vi "UI Main.vi"() -> ()   [LabVIEW 2020]
uses:
  controls/Control Configuration.ctl
  controls/UI Data.ctl
  controls/All Control Configuration Values.ctl
  controls/Control State.ctl
  controls/Raw Values.ctl
  Globals/Global - All UI Loop Stop.vi
  Globals/Global - UI Stream and Variable Connections.vi
  Globals/Global - Configuration Options.vi
  support/User Event - Stop/User Event - Stop.lvlib
  support/Message Queue/Message Queue.lvlib
panel:
  in  "Switch to Safe State":bool
  in  "Exit":bool
  out "System Status":string
  out "Current Control Mode":u16(ring) items=["Safe State", "Manual", "Control (PID)"]
  in  "Settings Tab":T1(tab)
  in  "Channel 3 Setpoint":dbl
  in  "Channel 2 Setpoint":dbl
  in  "Channel 1 Setpoint":dbl
  in  "Channel 0 Setpoint":dbl
  in  "Update Control Configuration":bool
  in  "Control Configurations":T2[](array[typedef])
  in  "Run Control":bool
  in  "Stop Control":bool
  in  "Channel 3 Manual Value":dbl
  in  "Channel 2 Manual Value":dbl
  in  "Channel 1 Manual Value":dbl
  in  "Channel 0 Manual Value":dbl
  in  "Run Manual":bool
  in  "Stop Manual":bool
  out "Control Input Values":T3(graph)
  out "Control Output Values":T3(graph)
  out "Control Loop Period (ms)":u32
  out "Largest Contiguous Memory (bytes)":dbl(graph)
  out "CPU Usage (%)":dbl(graph)
  out "Connected?":bool
  in  "Connect to Controller":bool
  in  "Controller Address":string
  # "LabVIEW Real-Time Control (NI-DAQmx)"
  # "Connection Settings"
  # "Element 0 - Chan 0\nElement 1 - Chan 1\nElement 2 - Chan 2\nElement 3 - Chan 3"
  # "Setpoint changes are sent to the target automatically."
  # "Control Configuration changes are sent to the target when you click \"Update Control Configurations\"."
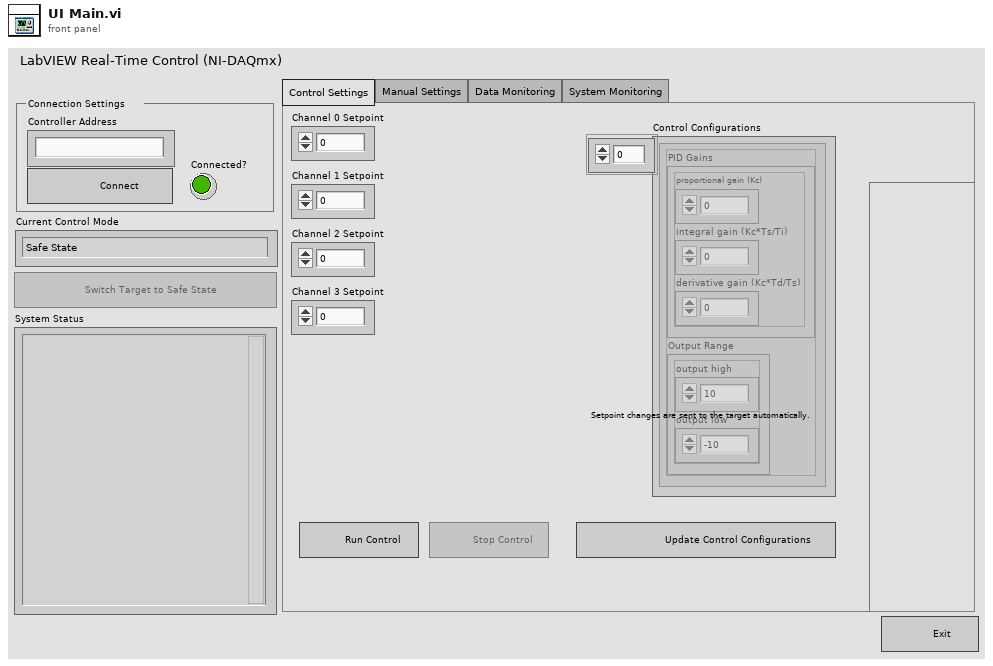
[diagram p1: front panel]
types:
  T1 = enum32{"Control Settings", "Manual Settings", "Data Monitoring", "System Monitoring"}
  T2 = typedef "Control Configuration.ctl" = cluster{"PID Gains":cluster{"proportional gain (Kc)":dbl, "integral gain (Kc*Ts/Ti)":dbl, "derivative gain (Kc*Td/Ts)":dbl}, "Output Range":cluster{"output high":dbl, "output low":dbl}}
  T3 = cluster{"Array of Double[0]":dbl, "Array of Double[1]":dbl, "Array of Double[2]":dbl, "Array of Double[3]":dbl}
  T4 = typedef "UI Data.ctl" = cluster{"Switch to Safe State Ref":refnum<vi>, "Run Manual Ref":refnum<vi>, "Stop Manual Ref":refnum<vi>, "Run Control Ref":refnum<vi>, "Stop Control Ref":refnum<vi>, "Update Control Configurations Ref":refnum<vi>, "Ch 0 Setpoint Ref":refnum<vi>, "Ch 1 Setpoint Ref":refnum<vi>, "Ch 2 Setpoint Ref":refnum<vi>, "Ch 3 Setpoint Ref":refnum<vi>, "Ch 0 Manual Ref":refnum<vi>, "Ch 1 Manual Ref":refnum<vi>, "Ch 2 Manual Ref":refnum<vi>, "Ch 3 Manual Ref":refnum<vi>, "Control Configurations Ref":refnum<vi>}
  T5 = typedef "Message Queue.lvlib/All Message Queues.ctl" = cluster{"UI":refnum<queue>}
  T6 = typedef "Variable References.ctl" = cluster{"CPU Usage":refnum<k21>, "Contiguous Memory":refnum<k21>, "Control Mode":refnum<k21>, "Control Loop Period":refnum<k21>, "Input Values":refnum<k21>, "Output Values":refnum<k21>}
  T7 = typedef "Control State.ctl" = enum16{"Safe State", "Manual", "Control (PID)"}
  T8 = cluster{"Channel 0 Setpoint":dbl, "Channel 1 Setpoint":dbl, "Channel 2 Setpoint":dbl, "Channel 3 Setpoint":dbl}
  T9 = cluster{"Channel 0 Manual Value":dbl, "Channel 1 Manual Value":dbl, "Channel 2 Manual Value":dbl, "Channel 3 Manual Value":dbl}
  T10 = cluster{"Message":string, "Message Data":variant}
  T11 = typedef "All Control Configuration Values.ctl" = cluster{"Control State":T7, "Setpoints":T12, "Manual Values":T12, "Control Configurations":T2[]}
  T12 = typedef "Raw Values.ctl" = cluster{"Channel 0":dbl, "Channel 1":dbl, "Channel 2":dbl, "Channel 3":dbl}
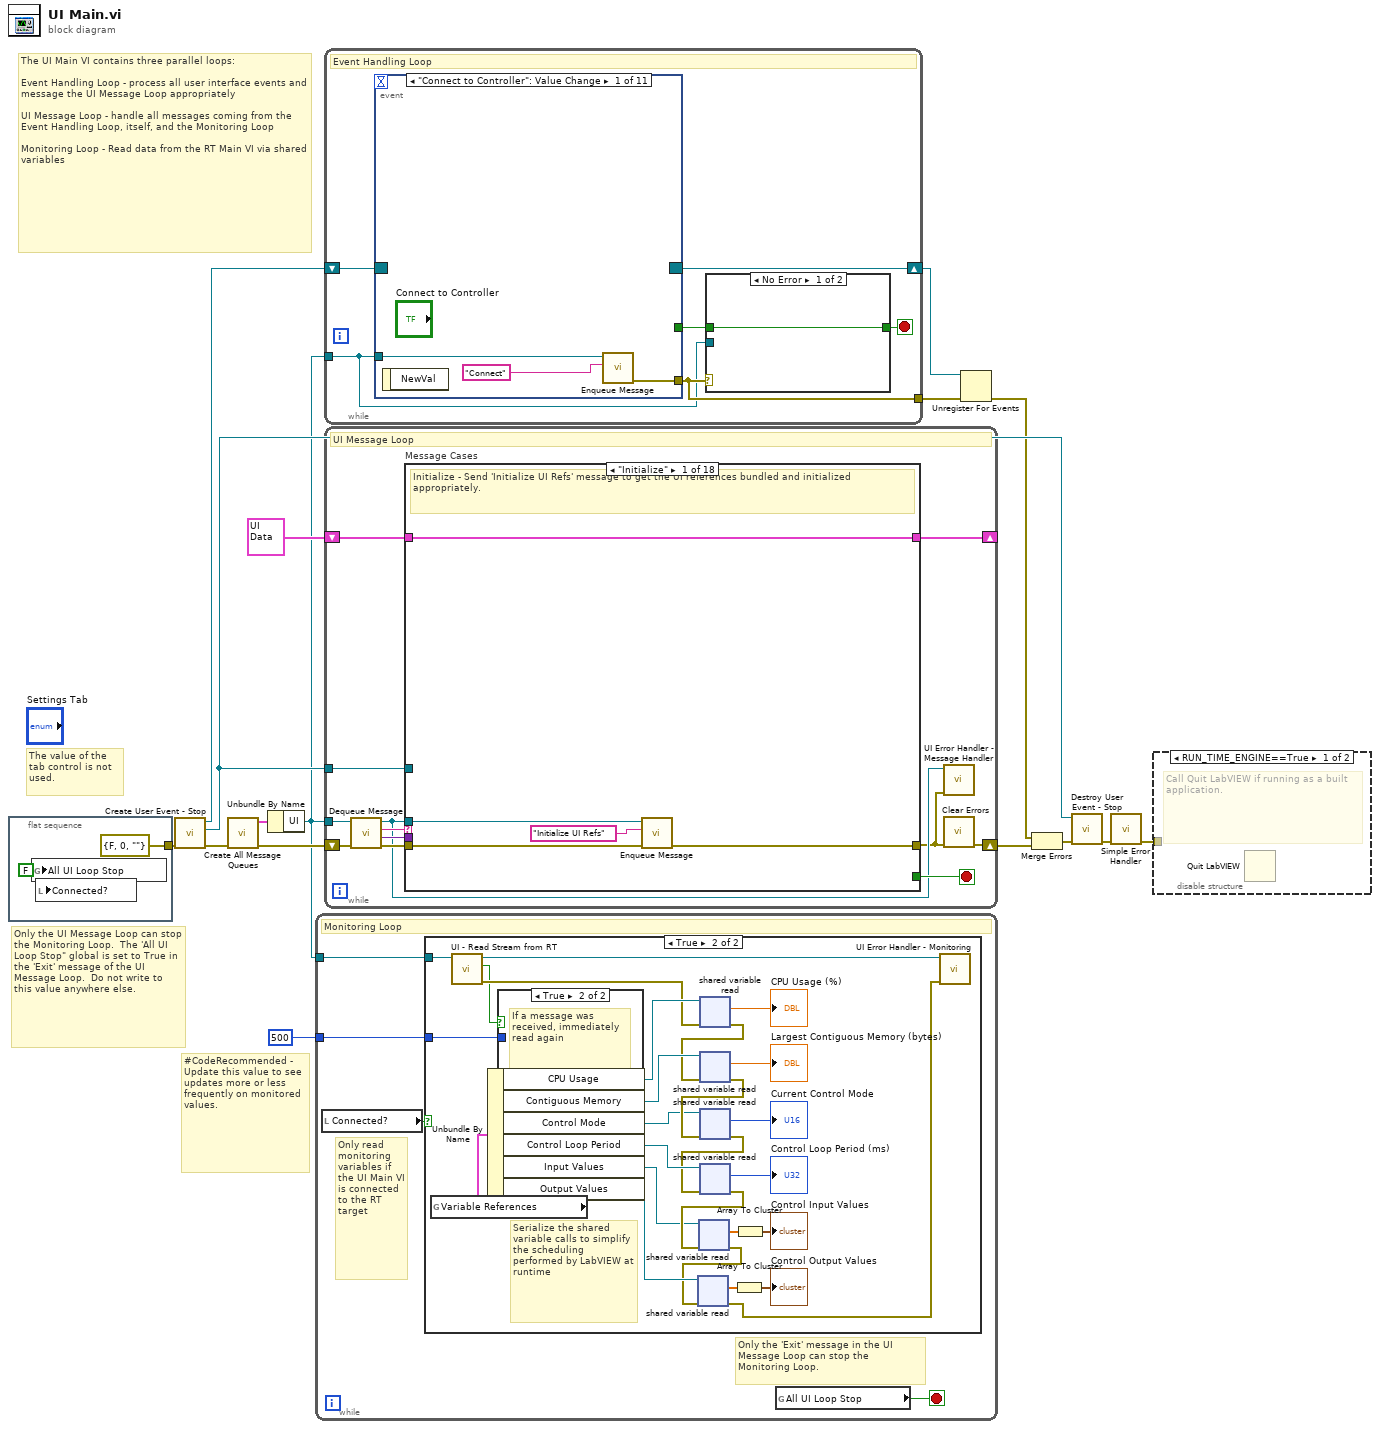
[diagram p0: block diagram]
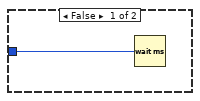
[diagram p3: hidden frame]
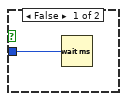
[diagram p4: hidden frame]
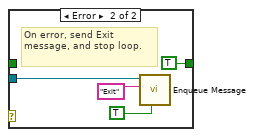
[diagram p5: hidden frame]
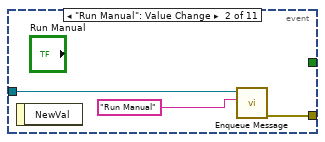
[diagram p6: hidden frame]
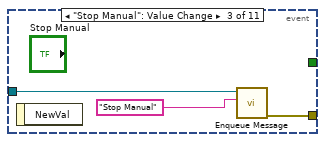
[diagram p7: hidden frame]
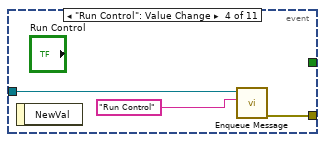
[diagram p8: hidden frame]
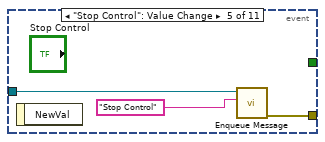
[diagram p9: hidden frame]
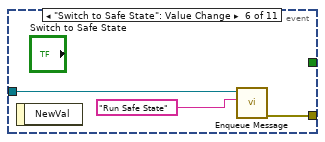
[diagram p10: hidden frame]
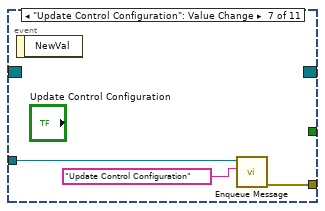
[diagram p11: hidden frame]
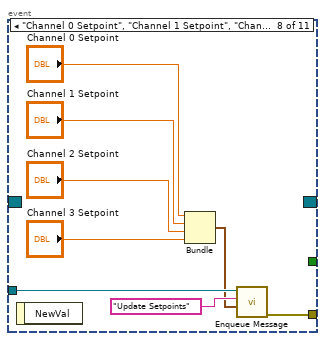
[diagram p12: hidden frame]
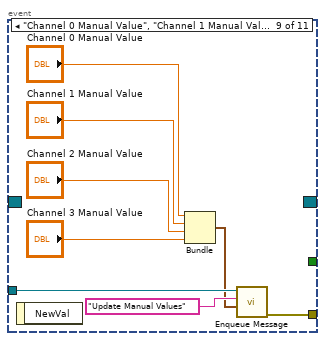
[diagram p13: hidden frame]
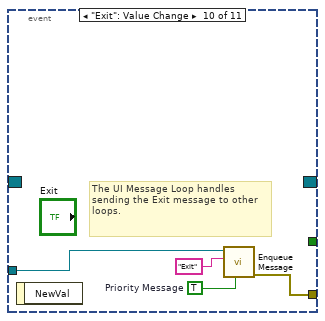
[diagram p14: hidden frame]
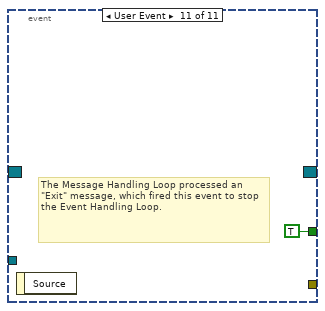
[diagram p15: hidden frame]
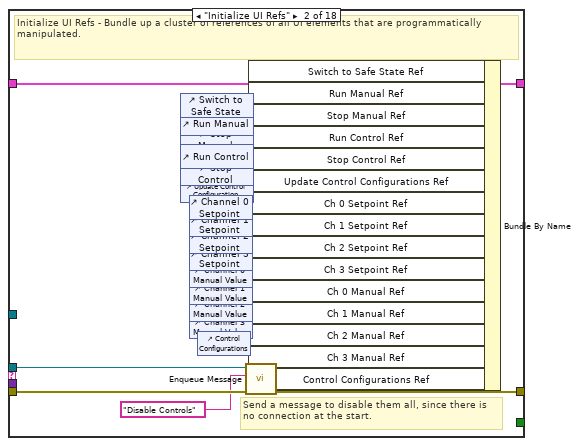
[diagram p16: hidden frame]
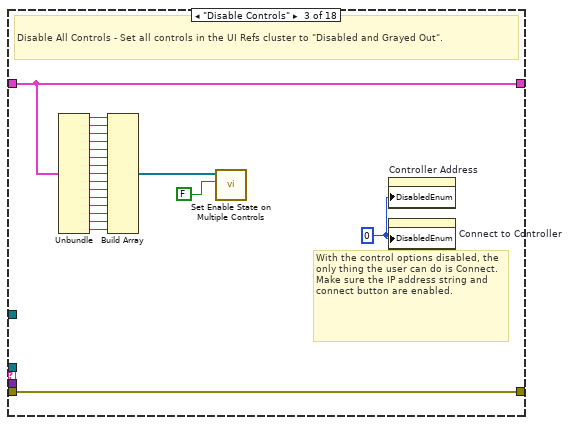
[diagram p17: hidden frame]
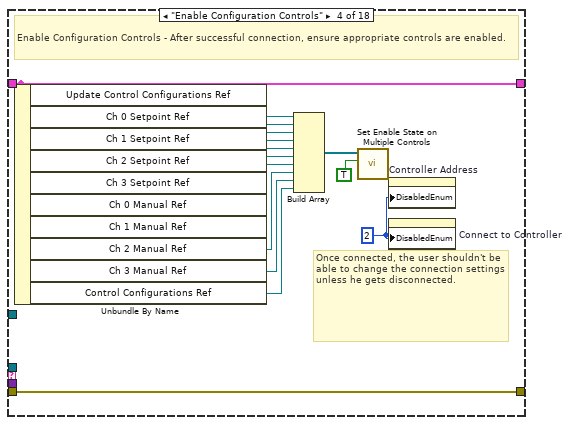
[diagram p18: hidden frame]
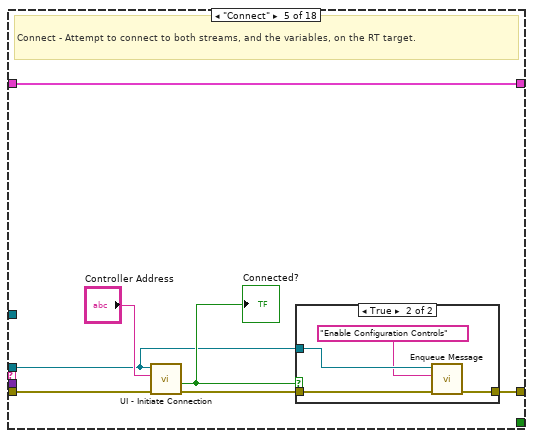
[diagram p19: hidden frame]
diagram:
  # "#CodeRecommended - Update this value to see updates more or less frequently on monitored values."
  # "The UI Main VI contains three parallel loops:\n\nEvent Handling Loop - process all user interface events and message the UI Message Loop appropriately\n\nUI Message Loop - handle all messages coming from the Event Handling Loop, itself, and the Monitoring Loop\n\nMonitoring Loop - Read data from the RT Main VI via shared variables"
  # "The value of the tab control is not used."
  # "Only the UI Message Loop can stop the Monitoring Loop.  The 'All UI Loop Stop\" global is set to True in the 'Exit' message of the UI Message Loop.  Do not write to this value anywhere else."
  n1 = flat-sequence {
    tunnel: [errorcluster {"status"=FALSE, "code"=0, "source"=""} ("error in (no error)")] -> w3
    frame #0 {
      w17 = FALSE
      n2 = global write "Global - All UI Loop Stop.vi" "All UI Loop Stop"(w17) -> ()
      n3 = local write "Connected?"(w17) -> ()
    }
  }
  n4 = call "Create User Event - Stop.vi"("error in (no error)"=w3) -> ("error out"=w11:errorcluster, "User Event - Stop"=w12:refnum<user-event>, "Stop Event Registration Refnum"=w13:refnum<event-registration>)  [unwired: 8 in]
  n5 = call "Create All Message Queues.vi"("error in (no error)"=w11) -> ("error out"=w9:errorcluster, "Message Queues out"=w10:T5)  [unwired: 9 in]
  n6 = Unbundle By Name(w10) -> ("UI"=w4:refnum<queue>)
  n7 = while {
    tunnel: w4 -> [w21]
    tunnel: u32 500 ("milliseconds to wait") -> [w19]
    stop <- w22 stop-if-true
    # "Only read monitoring variables if the UI Main VI is connected to the RT target"
    # "Only the 'Exit' message in the UI Message Loop can stop the Monitoring Loop."
    # "Monitoring Loop"
    n8 = local read "Connected?"() -> (w20:bool)
    n9 = case shown="True" w20 {
      tunnel: w21 -> [_ w40]
      tunnel: w19 -> [w23 w35]
      frame False {
        n10 = Wait (ms)(milliseconds to wait=w23) -> ()  [unwired: 1 out]
      }
      frame True {
        # "Serialize the shared variable calls to simplify the scheduling performed by LabVIEW at runtime"
        n11 = global read "Global - UI Stream and Variable Connections.vi" "Variable References"() -> (w38:T6)
        n12 = call "UI - Read Stream from RT.vi"("Message Queue"=w40) -> ("error out"=w43:errorcluster, "Message Received?"=w36:bool, "dup Message Queue"=w39:refnum<queue>)  [unwired: 8 in]
        n13 = Unbundle By Name(w38) -> ("CPU Usage"=w46:refnum<k21>, "Contiguous Memory"=w45:refnum<k21>, "Control Mode"=w33:refnum<k21>, "Control Loop Period"=w44:refnum<k21>, "Input Values"=w31:refnum<k21>, "Output Values"=w29:refnum<k21>)
        n14 = case shown="True" w36 {
          tunnel: w35 -> [w50 _]
          frame False {
            n15 = Wait (ms)(milliseconds to wait=w50) -> ()  [unwired: 1 out]
          }
          frame True {
            # "If a message was received, immediately read again"
          }
        }
        n16 = shared-variable-read(w46, w43) -> (w42:errorcluster, →"CPU Usage (%)":dbl)  [unwired: 2 out]
        n17 = shared-variable-read(w45, w42) -> (w34:errorcluster, →"Largest Contiguous Memory (bytes)":dbl)  [unwired: 2 out]
        n18 = shared-variable-read(w33, w34) -> (w41:errorcluster, →"Current Control Mode":T7)  [unwired: 2 out]
        n19 = shared-variable-read(w44, w41) -> (w32:errorcluster, →"Control Loop Period (ms)":u32)  [unwired: 2 out]
        n20 = shared-variable-read(w31, w32) -> (w28:errorcluster, w30:dbl[])  [unwired: 2 out]
        n21 = shared-variable-read(w29, w28) -> (w26:errorcluster, w27:dbl[])  [unwired: 2 out]
        n22 = Array To Cluster(array=w27) -> (cluster=→"Control Output Values":T3)
        n23 = Array To Cluster(array=w30) -> (cluster=→"Control Input Values":T3)
        n24 = call "UI Error Handler - Monitoring.vi"("error in (no error)"=w26, "Message Queue"=w39) -> ()  [unwired: 9 in, 1 out]
      }
    }
    n25 = global read "Global - All UI Loop Stop.vi" "All UI Loop Stop"() -> (w22:bool)
  }
  n26 = while {
    tunnel: w4 -> [w52]
    tunnel: [w54] -> w15
    shift-right: [w51] -> w7
    shift-left: w13 -> [w53]
    stop <- w55 stop-if-true
    # "Event Handling Loop"
    n27 = event shown="[0] \"Connect to Controller\": Value Change" {
      selector: w53 -> [_ _ _ _ _ _ _ _ _ _ _]
      dyn-events: [_ _ _ _ _ _ _ _ _ _ _] -> w51
      timeout: _ -> [_ _ _ _ _ _ _ _ _ _ _]
      tunnel: [_ _ _ _ _ _ _ _ _ _ TRUE ("Discard?")] -> w56
      tunnel: w52 -> [w62 w65 w68 w71 w74 w77 w82 w85 w97 w99 _]
      tunnel: [w64 w67 w70 w73 w76 w79 w81 w84 w96 w102 _] -> w54
      event "Connect to Controller": Value Change {
        n28 = event-data() -> ()  [unwired: 1 in, 1 out]
        n29 = call "Enqueue Message.vi"("Message"="Connect", "Message Queue"=w62) -> ("error out"=w64:errorcluster)  [unwired: 8 in, 1 out]
      }
      event "Run Manual": Value Change {
        n30 = event-data() -> ()  [unwired: 1 in, 1 out]
        n31 = call "Enqueue Message.vi"("Message"="Run Manual", "Message Queue"=w65) -> ("error out"=w67:errorcluster)  [unwired: 8 in, 1 out]
      }
      event "Stop Manual": Value Change {
        n32 = event-data() -> ()  [unwired: 1 in, 1 out]
        n33 = call "Enqueue Message.vi"("Message"="Stop Manual", "Message Queue"=w68) -> ("error out"=w70:errorcluster)  [unwired: 8 in, 1 out]
      }
      event "Run Control": Value Change {
        n34 = event-data() -> ()  [unwired: 1 in, 1 out]
        n35 = call "Enqueue Message.vi"("Message"="Run Control", "Message Queue"=w71) -> ("error out"=w73:errorcluster)  [unwired: 8 in, 1 out]
      }
      event "Stop Control": Value Change {
        n36 = event-data() -> ()  [unwired: 1 in, 1 out]
        n37 = call "Enqueue Message.vi"("Message"="Stop Control", "Message Queue"=w74) -> ("error out"=w76:errorcluster)  [unwired: 8 in, 1 out]
      }
      event "Switch to Safe State": Value Change {
        n38 = event-data() -> ()  [unwired: 1 in, 1 out]
        n39 = call "Enqueue Message.vi"("Message"="Run Safe State", "Message Queue"=w77) -> ("error out"=w79:errorcluster)  [unwired: 8 in, 1 out]
      }
      event "Update Control Configuration": Value Change {
        n40 = event-data() -> ()  [unwired: 1 in, 1 out]
        n41 = call "Enqueue Message.vi"("Message"="Update Control Configuration", "Message Queue"=w82) -> ("error out"=w81:errorcluster)  [unwired: 8 in, 1 out]
      }
      event "Channel 0 Setpoint", "Channel 1 Setpoint", "Channel 2 Setpoint", "Channel 3 Setpoint": Value Change {
        n42 = event-data() -> ()  [unwired: 1 in, 1 out]
        n43 = Bundle("Channel 0 Setpoint"="Channel 0 Setpoint", "Channel 1 Setpoint"="Channel 1 Setpoint", "Channel 2 Setpoint"="Channel 2 Setpoint", "Channel 3 Setpoint"="Channel 3 Setpoint") -> (w83:T8)  [unwired: 1 in]
        n44 = call "Enqueue Message.vi"("Message Data"=w83, "Message"="Update Setpoints", "Message Queue"=w85) -> ("error out"=w84:errorcluster)  [unwired: 7 in, 1 out]
      }
      event "Channel 0 Manual Value", "Channel 1 Manual Value", "Channel 2 Manual Value", "Channel 3 Manual Value": Value Change {
        n45 = event-data() -> ()  [unwired: 1 in, 1 out]
        n46 = Bundle("Channel 0 Manual Value"="Channel 0 Manual Value", "Channel 1 Manual Value"="Channel 1 Manual Value", "Channel 2 Manual Value"="Channel 2 Manual Value", "Channel 3 Manual Value"="Channel 3 Manual Value") -> (w95:T9)  [unwired: 1 in]
        n47 = call "Enqueue Message.vi"("Message Data"=w95, "Message"="Update Manual Values", "Message Queue"=w97) -> ("error out"=w96:errorcluster)  [unwired: 7 in, 1 out]
      }
      event "Exit": Value Change {
        w100 = TRUE  # Priority Message
        # "The UI Message Loop handles sending the Exit message to other loops."
        n48 = event-data() -> ()  [unwired: 1 in, 1 out]
        n49 = call "Enqueue Message.vi"("Priority Message? (F)"=w100, "Message"="Exit", "Message Queue"=w99) -> ("error out"=w102:errorcluster)  [unwired: 7 in, 1 out]
      }
      event User Event {
        # "The Message Handling Loop processed an \"Exit\" message, which fired this event to stop the Event Handling Loop."
        n50 = event-data() -> ()  [unwired: 1 in, 1 out]
      }
    }
    n51 = case shown="No Error" w54 {
      tunnel: [w57 TRUE ("Discard?")] -> w55
      tunnel: w56 -> [w57 _]
      tunnel: w52 -> [_ w58]
      frame No Error {
      }
      frame Error {
        # "On error, send Exit message, and stop loop."
        n52 = call "Enqueue Message.vi"("Priority Message? (F)"=TRUE ("Discard?"), "Message"="Exit", "Message Queue"=w58) -> ()  [unwired: 7 in, 2 out]
      }
    }
  }
  n53 = while {
    tunnel: w4 -> [w109]
    tunnel: w12 -> [w114]
    shift-right: [w104] -> w16
    shift-left: w9 -> [w113]
    shift-right: [w107] -> _
    shift-left: T4 {"Switch to Safe State Ref"=refnum, "Run Manual Ref"=refnum, "Stop Manual Ref"=refnum, "Run Control Ref"=refnum, "Stop Control Ref"=refnum, "Update Control Configurations Ref"=refnum, "Ch 0 Setpoint Ref"=refnum, "Ch 1 Setpoint Ref"=refnum, "Ch 2 Setpoint Ref"=refnum, "Ch 3 Setpoint Ref"=refnum, "Ch 0 Manual Ref"=refnum, "Ch 1 Manual Ref"=refnum, "Ch 2 Manual Ref"=refnum, "Ch 3 Manual Ref"=refnum, "Control Configurations Ref"=refnum} ("Measurement UI Controls") -> [w108]
    stop <- w115 stop-if-true
    # "UI Message Loop"
    n54 = call "Dequeue Message.vi"("error in (no error)"=w113, "Message Queue"=w109) -> ("error out"=w112:errorcluster, "Message Data"=w110:variant, "Message"=w111:string, "dup Message Queue"=w106:refnum<queue>)  [unwired: 6 in]
    n55 = case "Message Cases" shown="\"Initialize\"" w111 {
      selector: w111 -> [_ _ _ _ _ _ _ _ _ w238 _ w270 _ w320 _ _ _ w382]
      tunnel: w106 -> [w117 w129 _ _ w178 _ w196 _ w220 w239 _ _ _ w324 _ w367 _ _]
      tunnel: w112 -> [w119 w141 w161 w167 w183 w194 w198 w203 w234 w241 w259 w271 w284 w334 w355 w372 w377 _]
      tunnel: [w118 w130 w161 w167 w177 w194 w197 w202 w222 w240 w258 w272 w282 w335 w353 w373 w376 w380] -> w105
      tunnel: [_ _ _ _ _ _ _ _ _ _ _ _ _ _ _ TRUE _ _] -> w115
      tunnel: w110 -> [_ _ _ _ _ _ _ _ w232 _ _ w269 w283 w332 w352 _ _ _]
      tunnel: w114 -> [_ _ _ _ _ _ _ _ _ _ _ _ _ _ _ w371 _ _]
      tunnel: w108 -> [w120 w140 w160 w173 w182 w193 w200 w204 w229 w242 w260 w273 w281 w336 w354 w369 w375 w378]
      tunnel: [w120 w139 w160 w173 w182 w193 w200 w204 w229 w242 w260 w273 w281 w336 w354 w369 w375 w378] -> w107
      frame "Initialize" {
        # "Initialize - Send 'Initialize UI Refs' message to get the UI references bundled and initialized appropriately."
        n56 = call "Enqueue Message.vi"("error in (no error)"=w119, "Message"="Initialize UI Refs", "Message Queue"=w117) -> ("error out"=w118:errorcluster)  [unwired: 7 in, 1 out]
      }
      frame "Initialize UI Refs" {
        # "Send a message to disable them all, since there is no connection at the start."
        # "Initialize UI Refs - Bundle up a cluster of references of all UI elements that are programmatically manipulated."
        n57 = control-ref of="Switch to Safe State"() -> (w138:refnum<vi>)
        n58 = control-ref of="Run Manual"() -> (w122:refnum<vi>)
        n59 = control-ref of="Stop Manual"() -> (w121:refnum<vi>)
        n60 = control-ref of="Run Control"() -> (w137:refnum<vi>)
        n61 = control-ref of="Stop Control"() -> (w136:refnum<vi>)
        n62 = control-ref of="Update Control Configuration"() -> (w135:refnum<vi>)
        n63 = control-ref of="Channel 0 Setpoint"() -> (w134:refnum<vi>)
        n64 = control-ref of="Channel 1 Setpoint"() -> (w133:refnum<vi>)
        n65 = control-ref of="Channel 2 Setpoint"() -> (w132:refnum<vi>)
        n66 = control-ref of="Channel 3 Setpoint"() -> (w131:refnum<vi>)
        n67 = control-ref of="Channel 0 Manual Value"() -> (w126:refnum<vi>)
        n68 = control-ref of="Channel 1 Manual Value"() -> (w125:refnum<vi>)
        n69 = control-ref of="Channel 2 Manual Value"() -> (w124:refnum<vi>)
        n70 = control-ref of="Channel 3 Manual Value"() -> (w123:refnum<vi>)
        n71 = control-ref of="Control Configurations"() -> (w127:refnum<vi>)
        n72 = call "Enqueue Message.vi"("error in (no error)"=w141, "Message"="Disable Controls", "Message Queue"=w129) -> ("error out"=w130:errorcluster)  [unwired: 7 in, 1 out]
        n73 = Bundle By Name(cluster=w140, "Switch to Safe State Ref"=w138, "Run Manual Ref"=w122, "Stop Manual Ref"=w121, "Run Control Ref"=w137, "Stop Control Ref"=w136, "Update Control Configurations Ref"=w135, "Ch 0 Setpoint Ref"=w134, "Ch 1 Setpoint Ref"=w133, "Ch 2 Setpoint Ref"=w132, "Ch 3 Setpoint Ref"=w131, "Ch 0 Manual Ref"=w126, "Ch 1 Manual Ref"=w125, "Ch 2 Manual Ref"=w124, "Ch 3 Manual Ref"=w123, "Control Configurations Ref"=w127) -> (w139:T4)
      }
      frame "Disable Controls" {
        w148 = 0
        # "With the control options disabled, the only thing the user can do is Connect. Make sure the IP address string and connect button are enabled."
        # "Disable All Controls - Set all controls in the UI Refs cluster to \"Disabled and Grayed Out\"."
        n74 = Unbundle(w160) -> ("Switch to Safe State Ref"=w159:refnum<vi>, "Run Manual Ref"=w158:refnum<vi>, "Stop Manual Ref"=w157:refnum<vi>, "Run Control Ref"=w156:refnum<vi>, "Stop Control Ref"=w155:refnum<vi>, "Update Control Configurations Ref"=w154:refnum<vi>, "Ch 0 Setpoint Ref"=w153:refnum<vi>, "Ch 1 Setpoint Ref"=w152:refnum<vi>, "Ch 2 Setpoint Ref"=w151:refnum<vi>, "Ch 3 Setpoint Ref"=w147:refnum<vi>, "Ch 0 Manual Ref"=w146:refnum<vi>, "Ch 1 Manual Ref"=w145:refnum<vi>, "Ch 2 Manual Ref"=w144:refnum<vi>, "Ch 3 Manual Ref"=w143:refnum<vi>, "Control Configurations Ref"=w142:refnum<vi>)
        n75 = Build Array(w159, w158, w157, w156, w155, w154, w153, w152, w151, w147, w146, w145, w144, w143, w142) -> (w150:refnum<vi>[])
        n76 = call "Set Enable State on Multiple Controls.vi"("Enable?"=FALSE, "Controls"=w150) -> ()  [unwired: 10 in]
        n77 = property on="Controller Address" class="Str"("DisabledEnum"=w148) -> ()  [unwired: 2 in, 2 out]
        n78 = property on="Connect to Controller" class="Bool"("DisabledEnum"=w148) -> ()  [unwired: 2 in, 2 out]
      }
      frame "Enable Configuration Controls" {
        w174 = 2
        # "Once connected, the user shouldn't be able to change the connection settings unless he gets disconnected."
        # "Enable Configuration Controls - After successful connection, ensure appropriate controls are enabled."
        n79 = Unbundle By Name(w173) -> ("Update Control Configurations Ref"=w172:refnum<vi>, "Ch 0 Setpoint Ref"=w171:refnum<vi>, "Ch 1 Setpoint Ref"=w170:refnum<vi>, "Ch 2 Setpoint Ref"=w169:refnum<vi>, "Ch 3 Setpoint Ref"=w168:refnum<vi>, "Ch 0 Manual Ref"=w166:refnum<vi>, "Ch 1 Manual Ref"=w165:refnum<vi>, "Ch 2 Manual Ref"=w164:refnum<vi>, "Ch 3 Manual Ref"=w163:refnum<vi>, "Control Configurations Ref"=w162:refnum<vi>)
        n80 = Build Array(w172, w171, w170, w169, w168, w166, w165, w164, w163, w162) -> (w176:refnum<vi>[])
        n81 = call "Set Enable State on Multiple Controls.vi"("Enable?"=TRUE, "Controls"=w176) -> ()  [unwired: 10 in]
        n82 = property on="Controller Address" class="Str"("DisabledEnum"=w174) -> ()  [unwired: 2 in, 2 out]
        n83 = property on="Connect to Controller" class="Bool"("DisabledEnum"=w174) -> ()  [unwired: 2 in, 2 out]
      }
      frame "Connect" {
        # "Connect - Attempt to connect to both streams, and the variables, on the RT target."
        n84 = call "UI - Initiate Connection.vi"("error in (no error)"=w183, "Controller Address"="Controller Address", "Message Queue"=w178) -> ("error out"=w180:errorcluster, "Connected?"=w179:bool)  [unwired: 7 in]
        "Connected?" <- w179
        n85 = case shown="True" w179 {
          tunnel: w180 -> [w184 w188]
          tunnel: w178 -> [_ w187]
          tunnel: [w184 w186] -> w177
          frame False {
          }
          frame True {
            n86 = call "Enqueue Message.vi"("error in (no error)"=w188, "Message"="Enable Configuration Controls", "Message Queue"=w187) -> ("error out"=w186:errorcluster)  [unwired: 7 in, 1 out]
          }
        }
      }
      frame "Close Connections" {
        # "Close Connections - Close the connections shared with the Monitoring Loop."
        n87 = global read "Global - UI Stream and Variable Connections.vi" "UI Command Stream"() -> (w192:refnum<k21>)
        n88 = global read "Global - UI Stream and Variable Connections.vi" "Variable References"() -> (w190:T6)
        n89 = global read "Global - UI Stream and Variable Connections.vi" "RT Message Stream"() -> (w191:refnum<k21>)
        n90 = local write "Connected?"(FALSE ("Connected?")) -> ()
        n91 = Destroy Stream Endpoint(11:w192) -> ()  [unwired: 1 in, 1 out]
        n92 = Destroy Stream Endpoint(11:w191) -> ()  [unwired: 1 in, 1 out]
        n93 = call "Close Variable Connections.vi"("Variable References"=w190) -> ()  [unwired: 11 in]
      }
      frame "Disconnect UI" {
        # "Disconnect UI - Something has gone wrong with the connection. Reinitialize the UI to its disconnected state."
        n94 = local write "Connected?"(FALSE ("Connected?")) -> ()
        n95 = call "Enqueue Message.vi"("error in (no error)"=w198, "Message"="Disable Controls", "Message Queue"=w196) -> ("error out"=w197:errorcluster)  [unwired: 7 in, 1 out]
      }
      frame "Get Control Settings from RT" {
        # "Get Control Settings from RT - Send a command to the RT to retrieve all current control parameter values and send them back to the UI."
        n96 = local read "Connected?"() -> (w201:bool)
        n97 = case shown="True" w201 {
          tunnel: w203 -> [w205 w209]
          tunnel: [w205 w208] -> w202
          frame False {
            # "Don't bother trying to send a message to the RT system if UI Main VI isn't even connected"
          }
          frame True {
            n98 = global read "Global - UI Stream and Variable Connections.vi" "UI Command Stream"() -> (w206:refnum<k21>)
            n99 = shared-variable-write(w206, w209, T10 {"Message"="Send Control Configuration to UI", "Message Data"=variant} ("data in")) -> (w208:errorcluster)  [unwired: 1 in, 2 out]
          }
        }
      }
      frame "Initial UI Values" {
        # "Set values of all setpoint and manual controls via reference."
        # "Initial UI Values - These are the current control values from the RT Control Loop. They are used to initialize the panel of UI Main VI upon successful connection to the RT target."
        n100 = Unbundle By Name(w229) -> ("Ch 0 Setpoint Ref"=w228:refnum<vi>, "Ch 1 Setpoint Ref"=w227:refnum<vi>, "Ch 2 Setpoint Ref"=w226:refnum<vi>, "Ch 3 Setpoint Ref"=w225:refnum<vi>, "Ch 0 Manual Ref"=w218:refnum<vi>, "Ch 1 Manual Ref"=w217:refnum<vi>, "Ch 2 Manual Ref"=w216:refnum<vi>, "Ch 3 Manual Ref"=w215:refnum<vi>)
        n101 = Variant To Data(error in=w234, type=T11 {"Control State"=enum."Safe State", "Setpoints"={"Channel 0"=0.0, "Channel 1"=0.0, "Channel 2"=0.0, "Channel 3"=0.0}, "Manual Values"={"Channel 0"=0.0, "Channel 1"=0.0, "Channel 2"=0.0, "Channel 3"=0.0}, "Control Configurations"=[]} ("All FPGA Configuration Values"), Variant=w232) -> (data=w230:T11, error out=w233:errorcluster)
        n102 = Unbundle By Name(w230) -> ("Setpoints"=w214:T12, "Manual Values"=w213:T12, "Control Configurations"=w223:T2[], "Control State"=w219:T7)
        n103 = Build Array(w228, w227, w226, w225, w218, w217, w216, w215) -> (w224:refnum<vi>[])
        n104 = Cluster To Array(cluster=w214) -> (array=w212:dbl[])
        n105 = Cluster To Array(cluster=w213) -> (array=w211:dbl[])
        n106 = local write "Control Configurations"(w223) -> ()
        n107 = local write "Current Control Mode"(w219) -> ()
        n108 = Build Array (concatenate)(w212, w211) -> (w210:dbl[])
        n109 = for {
          tunnel: w224 -> [w236] mode=indexing
          tunnel: w210 -> [w235] mode=indexing
          n110 = property class="DigNum"(reference=w236, "Value"=w235) -> ()  [unwired: 1 in, 2 out]
        }
        n111 = call "Enqueue Message.vi"("error in (no error)"=w233, "Message Data"=w219, "Message"="Update Display Mode", "Message Queue"=w220) -> ("error out"=w222:errorcluster)  [unwired: 6 in, 1 out]
      }
      frame "Run Control", "Run Manual", "Run Safe State", "Stop Control", "Stop Manual" {
        # "Run/Stop buttons - Send a command to switch the RT control loop into the appropriate state. Send a message to update this UI to reflect the new state."
        n112 = local read "Connected?"() -> (w237:bool)
        n113 = case shown="True" w237 {
          tunnel: w241 -> [w243 w253]
          tunnel: [w243 w249] -> w240
          tunnel: w239 -> [_ w248]
          tunnel: w238 -> [_ w247]
          frame False {
            # "Don't bother trying to send a message to the RT system if UI Main VI isn't even connected"
          }
          frame True {
            # "Run Control switches into its respective states. Anything else switches to Safe State."
            n114 = case shown="\"Safe State\", \"Stop Control\", \"Stop Manual\", Default" w247 {
              tunnel: [Control_State."Safe State" ("FPGA State") Control_State."Control (PID)" ("FPGA State") Control_State."Manual" ("FPGA State")] -> w244
              frame "Safe State", "Stop Control", "Stop Manual", Default {
              }
              frame "Run Control" {
              }
              frame "Run Manual" {
              }
            }
            n115 = global read "Global - UI Stream and Variable Connections.vi" "UI Command Stream"() -> (w245:refnum<k21>)
            n116 = Bundle("Update Control State", "FPGA State"=w244) -> (w250:cluster{string, "FPGA State":T7})  [unwired: 1 in]
            n117 = shared-variable-write(w245, w253, w250) -> (w252:errorcluster)  [unwired: 1 in, 2 out]
            n118 = call "Enqueue Message.vi"("error in (no error)"=w252, "Message Data"=w244, "Message"="Update Display Mode", "Message Queue"=w248) -> ("error out"=w249:errorcluster)  [unwired: 6 in, 1 out]
          }
        }
      }
      frame "Update Control Configuration" {
        # "Update Control Configuration - Send all control configurations to RT."
        n119 = local read "Connected?"() -> (w257:bool)
        n120 = case shown="True" w257 {
          tunnel: w259 -> [w261 w267]
          tunnel: [w261 w266] -> w258
          frame False {
            # "Don't bother trying to send a message to the RT system if UI Main VI isn't even connected"
          }
          frame True {
            n121 = global read "Global - UI Stream and Variable Connections.vi" "UI Command Stream"() -> (w262:refnum<k21>)
            n122 = Bundle("Update Control Configurations", "Control Configurations"="Control Configurations") -> (w264:cluster{string, "Control Configurations":T2[]})  [unwired: 1 in]
            n123 = shared-variable-write(w262, w267, w264) -> (w266:errorcluster)  [unwired: 1 in, 2 out]
          }
        }
      }
      frame "Update Manual Values", "Update Setpoints" {
        # "Update Setpoints/Manual Values - Send all setpoints/manual values to RT."
        n124 = local read "Connected?"() -> (w268:bool)
        n125 = case shown="True" w268 {
          tunnel: [w274 w280] -> w272
          tunnel: w271 -> [w274 w278]
          tunnel: w270 -> [_ w277]
          tunnel: w269 -> [_ w276]
          frame False {
            # "Don't bother trying to send a message to the RT system if UI Main VI isn't even connected"
          }
          frame True {
            n126 = global read "Global - UI Stream and Variable Connections.vi" "UI Command Stream"() -> (w275:refnum<k21>)
            n127 = Bundle(w277, "Message Data"=w276) -> (w279:cluster{string, "Message Data":variant})  [unwired: 1 in]
            n128 = shared-variable-write(w275, w278, w279) -> (w280:errorcluster)  [unwired: 1 in, 2 out]
          }
        }
      }
      frame "Update Display Mode" {
        # "Update Display Mode - Enable/Disable Controls appropriately for the new display mode."
        n129 = Variant To Data(error in=w284, type=Control_State."Safe State" ("Control State"), Variant=w283) -> (data=w291:T7, error out=w282:errorcluster)
        n130 = Unbundle By Name(w281) -> ("Switch to Safe State Ref"=w290:refnum<vi>, "Run Manual Ref"=w289:refnum<vi>, "Stop Manual Ref"=w288:refnum<vi>, "Run Control Ref"=w287:refnum<vi>, "Stop Control Ref"=w286:refnum<vi>)
        n131 = case shown="\"Control (PID)\"" w291 {
          tunnel: w290 -> [w296 w305 w312]
          tunnel: w289 -> [w292 w304 w314]
          tunnel: w288 -> [w295 w303 w311]
          tunnel: w287 -> [w294 w301 w313]
          tunnel: w286 -> [w293 w302 w310]
          frame "Control (PID)" {
            n132 = Build Array "Controls to Enable"(w296, w293, w292) -> (w300:refnum<vi>[])
            n133 = Build Array "Controls to Disable"(w295, w294) -> (w298:refnum<vi>[])
            n134 = call "Set Enable State on Multiple Controls.vi"("Enable?"=FALSE, "Controls"=w298) -> ()  [unwired: 10 in]
            n135 = call "Set Enable State on Multiple Controls.vi"("Enable?"=TRUE, "Controls"=w300) -> ()  [unwired: 10 in]
          }
          frame "Manual" {
            n136 = Build Array "Controls to Enable"(w305, w303, w301) -> (w309:refnum<vi>[])
            n137 = Build Array "Controls to Disable"(w304, w302) -> (w307:refnum<vi>[])
            n138 = call "Set Enable State on Multiple Controls.vi"("Enable?"=FALSE, "Controls"=w307) -> ()  [unwired: 10 in]
            n139 = call "Set Enable State on Multiple Controls.vi"("Enable?"=TRUE, "Controls"=w309) -> ()  [unwired: 10 in]
          }
          frame "Safe State" {
            # "This frame runs when the Control loop is in Safe State. Only enable the two run buttons."
            n140 = Build Array "Controls to Enable"(w314, w313) -> (w318:refnum<vi>[])
            n141 = Build Array "Controls to Disable"(w312, w311, w310) -> (w316:refnum<vi>[])
            n142 = call "Set Enable State on Multiple Controls.vi"("Enable?"=FALSE, "Controls"=w316) -> ()  [unwired: 10 in]
            n143 = call "Set Enable State on Multiple Controls.vi"("Enable?"=TRUE, "Controls"=w318) -> ()  [unwired: 10 in]
          }
        }
      }
      frame "Critical Error", "Log-Only Error", "Non-Critical Error", "RT Error" {
        # "Error - Display message in status indicator on panel.  If it's a critical error, shut down this VI with an 'Exit' message."
        n144 = case shown="Default" w320 {
          selector: w320 -> [_ w338]
          tunnel: ["UI Error" w338] -> w319
          frame Default {
          }
          frame "RT Error" {
          }
        }
        n145 = Variant To Data(error in=w334, type=errorcluster {"status"=FALSE, "code"=0, "source"=""} ("error constant"), Variant=w332) -> (data=w327:errorcluster, error out=w333:errorcluster)
        n146 = Unbundle By Name(w327) -> ("code"=w326:i32, "source"=w330:string)
        n147 = Format Date/Time String() -> (date/time string=w329:string)  [unwired: 3 in]
        n148 = Format Into String(format string="\n%s: %s %d - %s", w329, w319, w326, w330) -> (resulting string=w321:string)  [unwired: 2 in, 1 out]
        n149 = call "Enqueue Message.vi"("error in (no error)"=w333, "Message Data"=w321, "Message"="Update System Status", "Message Queue"=w324) -> ("error out"=w325:errorcluster, "dup Message Queue"=w323:refnum<queue>)  [unwired: 6 in]
        n150 = case shown="Default" w320 {
          tunnel: w325 -> [w339 w343]
          tunnel: w323 -> [_ w341]
          tunnel: [w339 w342] -> w335
          frame Default {
          }
          frame "Critical Error" {
            n151 = call "Enqueue Message.vi"("error in (no error)"=w343, "Message"="Exit", "Message Queue"=w341) -> ("error out"=w342:errorcluster)  [unwired: 7 in, 1 out]
          }
        }
      }
      frame "Update System Status" {
        # "#CodeRecommended - The code below ensures that the System Status string value does not become too large.  It uses the same maximum size as the RT error log to determine whether or not to remove the last half of the log string. Change this logic if you wish to maintain more/less of the information in the System Status string."
        # "Update System Status - Add a new string to the beginning of the System Status string on the UI."
        n152 = Variant To Data(error in=w355, type="", Variant=w352) -> (data=w349:string, error out=w353:errorcluster)
        n153 = local read "System Status"() -> (w347:string)
        n154 = global read "Global - Configuration Options.vi" "Error Log Max Size (bytes)"() -> (w345:i64)
        n155 = String Length(string=w347) -> (length=w348:i32)
        n156 = Greater?(x=w348, y=w345) -> (0:w346:bool)
        n157 = case shown="True" w346 {
          tunnel: w347 -> [w356 w360]
          tunnel: w345 -> [_ w359]
          tunnel: [w356 w361] -> w344
          frame False {
          }
          frame True {
            n158 = Divide(x=w359, y=i64 2) -> (x/y=w358:dbl)
            n159 = String Subset(string=w360, length (rest)=w358) -> (substring=w361:string)  [unwired: 1 in]
          }
        }
        n160 = Concatenate Strings(w349, w344) -> (→"System Status":string)
      }
      frame "Exit" {
        # "Flush the Writer Stream to ensure all pending messages are sent to RT Main VI"
        # "Close all connections"
        # "Stop Monitoring Loop"
        # "Stop Event Handling Loop"
        # "Release the UI Message queue reference"
        # "Stop UI Message Loop"
        # "Exit - Fire the User Event to stop the Event Handling Loop, and toggle the global variable to stop the Monitoring Loop.  This message alone causes all three loops to stop."
        n161 = global write "Global - All UI Loop Stop.vi" "All UI Loop Stop"(TRUE ("Stop Monitoring Loop")) -> ()
        n162 = call "Fire User Event - Stop.vi"("User Event - Stop"=w371) -> ("error out"=w370:errorcluster)  [unwired: 10 in]
        n163 = Release Queue(queue=w367, error in (no error)=w372) -> (error out=w368:errorcluster)  [unwired: 1 in, 2 out]
        n164 = global read "Global - UI Stream and Variable Connections.vi" "UI Command Stream"() -> (w363:refnum<k21>)
        n165 = global read "Global - UI Stream and Variable Connections.vi" "Variable References"() -> (w364:T6)
        n166 = global read "Global - UI Stream and Variable Connections.vi" "RT Message Stream"() -> (w365:refnum<k21>)
        n167 = Flush Stream(11:w363) -> (3:w362:refnum<k21>)  [unwired: 3 in, 2 out]
        n168 = Destroy Stream Endpoint(11:w365) -> ()  [unwired: 1 in, 1 out]
        n169 = call "Close Variable Connections.vi"("Variable References"=w364) -> ()  [unwired: 11 in]
        n170 = Destroy Stream Endpoint(11:w362) -> ()  [unwired: 1 in, 1 out]
        n171 = Merge Errors(w370, w368) -> (w373:errorcluster)
      }
      frame "---Copy This Frame---" {
        # "Duplicate this frame when creating new messages.  Change this comment in the duplicated frame to describe this message."
        n172 = Merge Errors(w377) -> (w376:errorcluster)
      }
      frame Default {
        # "'Default' case only runs if there is a message that isn't defined in any of the other cases.  Output a programming error."
        n173 = Format Into String(format string="The invalid message string \"%s\" was received in the Message Handling Loop." ("Invalid Message Loop Message"), w382) -> (resulting string=w379:string)  [unwired: 2 in, 1 out]
        n174 = call <vilib>:"Error Cluster From Error Code.vi"("error message (\"\")"=w379, "error code (0)"=1) -> ("error out"=w380:errorcluster)  [unwired: 7 in]
      }
    }
    n175 = call "UI Error Handler - Message Handler.vi"("error in (no error)"=w105, "Message Queue"=w106) -> ()  [unwired: 9 in, 1 out]
    n176 = call <vilib>:"Clear Errors.vi"("error in (no error)"=w105) -> ("error out"=w104:errorcluster)  [unwired: 5 in, 1 out]
  }
  n177 = Unregister For Events(event registration refnum=w7, error in=w15) -> (error out=w8:errorcluster)
  n178 = Merge Errors(w8, w16) -> (w14:errorcluster)
  n179 = call "Destroy User Event - Stop.vi"("error in (no error)"=w14, "User Event - Stop"=w12) -> ("error out"=w5:errorcluster)  [unwired: 9 in]
  n180 = call <vilib>:"Simple Error Handler.vi"("error in (no error)"=w5) -> ("error out"=w1:errorcluster)  [unwired: 4 in, 4 out]
  n181 = disable-structure shown="RUN_TIME_ENGINE==True" {
    disable-tunnel: w1 -> [_ _]
    frame condition #0 {
      # "Call Quit LabVIEW if running as a built application."
      n182 = Quit LabVIEW() -> ()  [unwired: 1 in]
    }
    frame condition #1 (active) {
    }
  }
